vi "Process Outgoing Messages by Frame Type.vi"(0 "internal data":T1={"J1939 XNET Settings"={"XNET Database"="", "XNET Cluster"="", "CAN port"="", "Baud rate [Bd]"=0, "J1939 Network Address"=0, "Name"=0, "Termination"=0}, "j1939 queues"={"Processed Outgoing"=refnum, "Process Outgoing"=refnum, "stop notifier"=refnum, "error queue"=refnum, "active dtc"=refnum, "processed inc"=refnum}, "fgv references"={"BAM Buffer"=refnum, "CM Buffer"=refnum, "CM Gen"=refnum, "BAM Gen"=refnum, "Address Claims"=refnum, "RQST"=refnum, "scaling lut"=refnum, "data lut"=refnum, "cyclic scheduler"=refnum}, "frame in"="", "frame out"="", "timing"={"tb to j1939 queue timeout"=100, "j1939 to tb queue timeout"=100, "dtc loop period (ms)"=100, "CAN in loop period (ms)"=100, "process incoming queue timeout (ms)"=100, "Outgoing Write Decimation"=0, "process outgoing loop rate (ms)"=0, "periodic outgoing queue timeout (ms)"=10, "CAN out queue timeout (ms)"=100}}, 5 "Output Array":T14[](array[typedef]) {"Identifier" format="%08x"}, 11 "error in":errorcluster) -> (13 "Message Errors":errorcluster, 15 "System Error":errorcluster)   [LabVIEW 2013, in "J1939.lvlib"]
uses:
  J1939.lvlib
  API Types/CAN Outgoing Message Cluster.ctl
  API Types/Internal Data.ctl
  API Types/XNET Settings.ctl
  API Types/Setup Information Cluster.ctl
  API Types/Convert DTCs Cluster.ctl
  <vilib>/xnet/xnet.llb/XNET Frame CAN.ctl
  <vilib>/xnet/xnet.llb/XNET Frame Type CAN.ctl
  TP/TP List References.ctl
  BAM/BAM Buffer Connections List_Ref.ctl
  Connection Mode/Connection Mode Generation Connection Ref.ctl
  BAM/BAM Generation Connections List_Ref.ctl
  LUTs/J1939 Address Table Reference.ctl
  RQST/RQST Lookup Table Reference.ctl
  LUTs/J1939 Conversion Lookup Table Reference.ctl
  LUTs/J1939 Data Lookup Table Reference.ctl
  LUTs/Cyclic Frame Scheduler Lut Reference.ctl
  Configuration/TypeDefs/timing configuration.ctl
  TP/TP Connections List State.ctl
  BAM/BAM Generation Connections List_Actions.vi
  BAM/BAM Generation Create New TP Connection.vi
  Connection Mode/Connection Mode Generation Connections List_Actions.vi
  Connection Mode/Connection Mode Generation Search for Connection (Local Message).vi
  Connection Mode/Connection Mode Generation Create New TP Connection.vi
  Frame Conversion/Common Conversions.vi
  Frame Conversion/Convert CAN Arb ID to J1939 ID.vi
  Common Messages/J1939 Common Messages.vi
  Common Messages/J1939 Message TP.CM BAM.vi
  Common Messages/J1939 Message TP.DT.vi
  Common Messages/J1939 Message TP.CM RTS.vi
  Frame Conversion/Convert J1939 ID to CAN Arb ID.vi
  BAM/BAM Generation Search for Connection (Local Message).vi
panel:
  in  "Allow Any Source Address":bool=TRUE
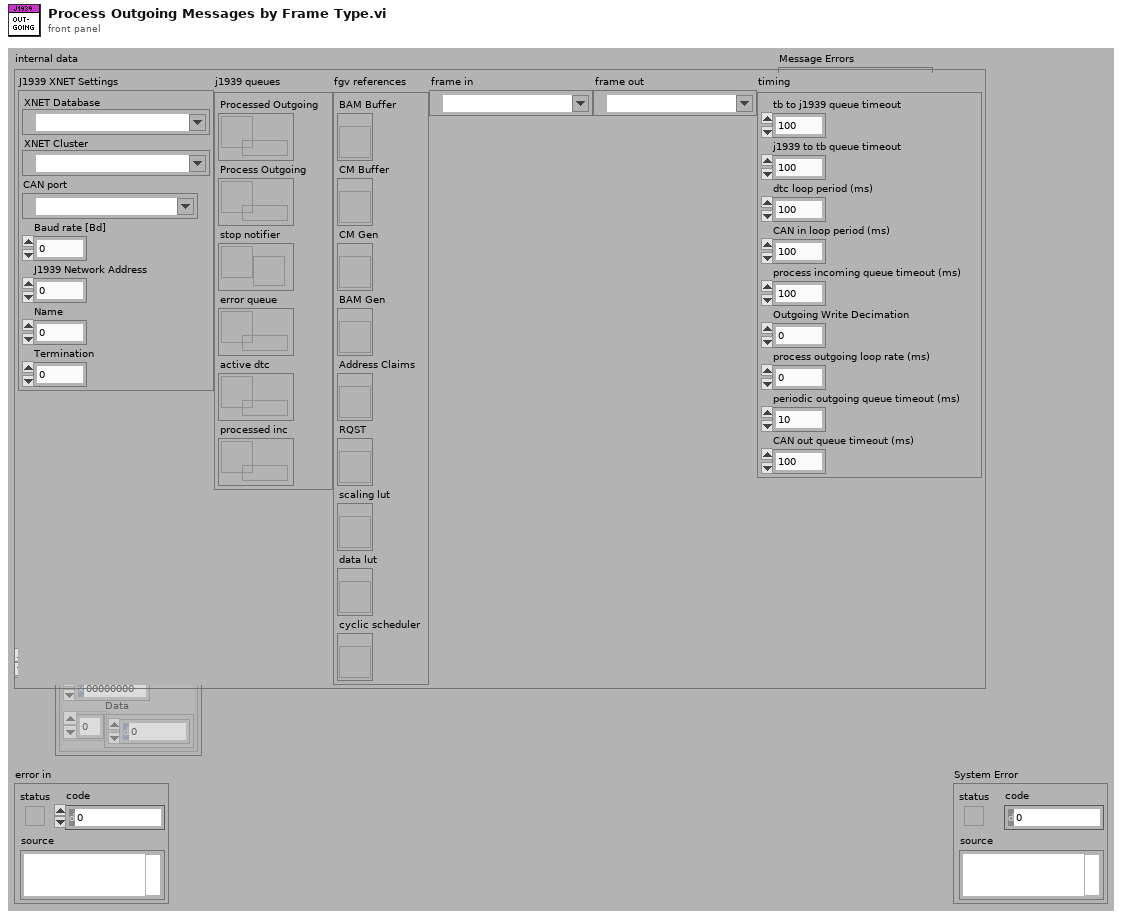
[diagram p1: front panel]
types:
  T1 = typedef "J1939.lvlib/Internal Data.ctl" = cluster{"J1939 XNET Settings":T2, "j1939 queues":T3, "fgv references":T4, "frame in":refnum<k21>, "frame out":refnum<k21>, "timing":T13}
  T2 = typedef "J1939.lvlib/XNET settings.ctl" = cluster{"XNET Database":refnum<k21>, "XNET Cluster":refnum<k21>, "CAN port":refnum<k21>, "Baud rate [Bd]":u32, "J1939 Network Address":u8, "Name":u64, "Termination":u32}
  T3 = typedef "J1939.lvlib/Setup Information Cluster.ctl" = cluster{"Processed Outgoing":refnum<queue>, "Process Outgoing":refnum<queue>, "stop notifier":refnum<notifier>, "error queue":refnum<queue>, "active dtc":refnum<queue>, "processed inc":refnum<queue>}
  T4 = typedef "J1939.lvlib/TP List References.ctl" = cluster{"BAM Buffer":T5, "CM Buffer":T5, "CM Gen":T6, "BAM Gen":T7, "Address Claims":T8, "RQST":T9, "scaling lut":T10, "data lut":T11, "cyclic scheduler":T12}
  T5 = typedef "J1939.lvlib/BAM Buffer Connections List_Ref.ctl" = refnum<vi>
  T6 = typedef "J1939.lvlib/Connection Mode Generation Connection Ref.ctl" = refnum<vi>
  T7 = typedef "J1939.lvlib/BAM Generation Connections List_Ref.ctl" = refnum<vi>
  T8 = typedef "J1939.lvlib/J1939 Address Table Reference.ctl" = refnum<vi>
  T9 = typedef "J1939.lvlib/RQST Lookup Table Reference.ctl" = refnum<vi>
  T10 = typedef "J1939.lvlib/J1939 Conversion Lookup Table Reference.ctl" = refnum<vi>
  T11 = typedef "J1939.lvlib/J1939 Data Lookup Table Reference.ctl" = refnum<vi>
  T12 = typedef "J1939.lvlib/cyclic frame scheduler lut reference.ctl" = refnum<vi>
  T13 = typedef "J1939.lvlib/timing configuration.ctl" = cluster{"tb to j1939 queue timeout":i32, "j1939 to tb queue timeout":i32, "dtc loop period (ms)":i32, "CAN in loop period (ms)":i32, "process incoming queue timeout (ms)":i32, "Outgoing Write Decimation":u32, "process outgoing loop rate (ms)":i32, "periodic outgoing queue timeout (ms)":i32, "CAN out queue timeout (ms)":i32}
  T14 = typedef "J1939.lvlib/CAN Outgoing Message Cluster.ctl" = cluster{"Identifier":u32, "Data":u8[]}
  T15 = typedef "J1939.lvlib/TP Connections List State.ctl" = enum16{"Add", "Update", "Get", "Remove", "Initialize"}
  T16 = typedef "J1939.lvlib/Outgoing Messages Frame Type.ctl" = enum16{"Standard Frame", "BAM", "Connection Mode"}
  T17 = typedef "J1939.lvlib/BAM Generation Connection Cluster.ctl" = cluster{"Total Packets":u8, "Current Packet to Generate":u8, "Packets":T14[], "Previous Time Stamp":u32, "Total Bytes":u16, "Source Address":u8}
  T18 = typedef "J1939.lvlib/Connection Mode Generation Connection Cluster.ctl" = cluster{"Total Packets":u8, "Current Packet to Generate":u8, "Packets":T14[], "Previous Time Stamp":u32, "Total Bytes":u16, "Packet Identifier [PDU S + SA]":u16, "Number of Packets to Generate":u8, "PGN":u32}
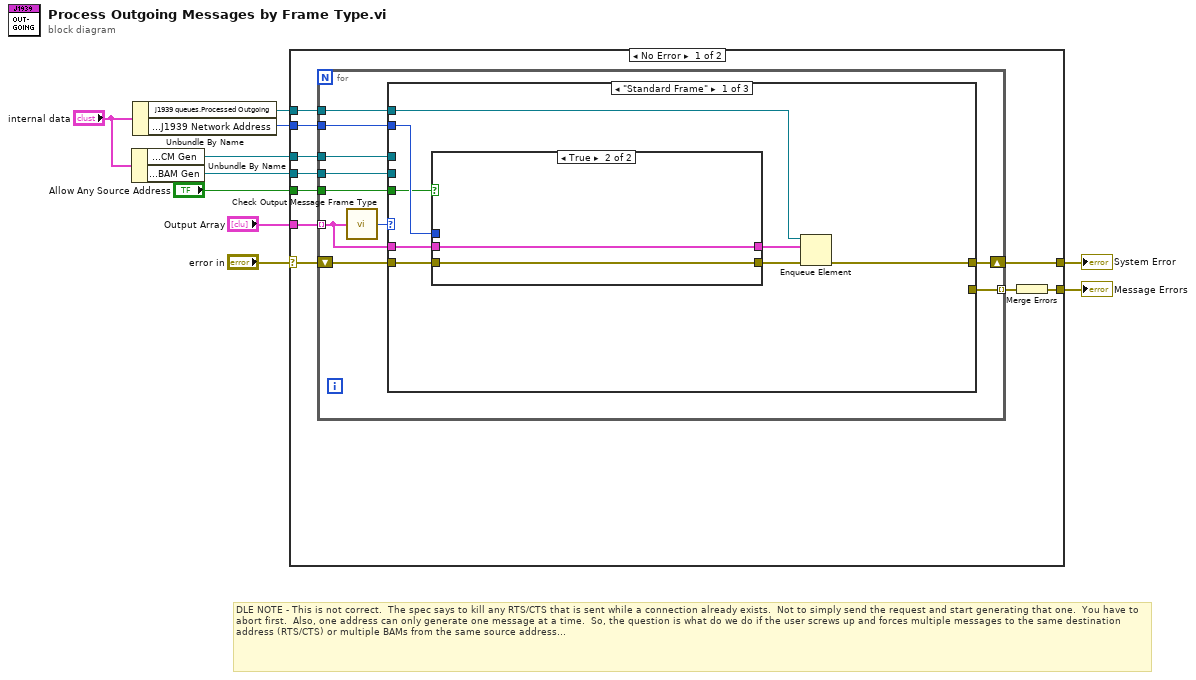
[diagram p0: block diagram]
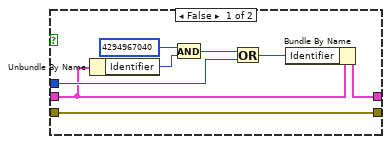
[diagram p2: hidden frame]
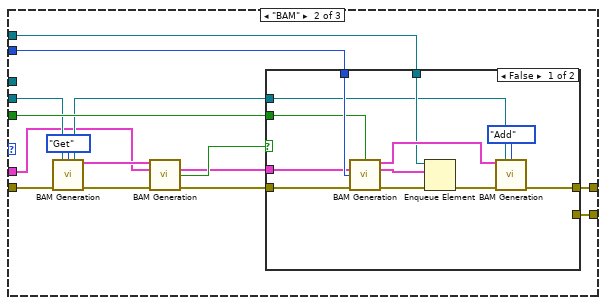
[diagram p3: hidden frame]
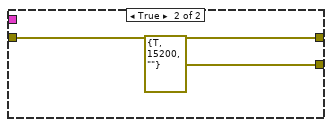
[diagram p4: hidden frame]
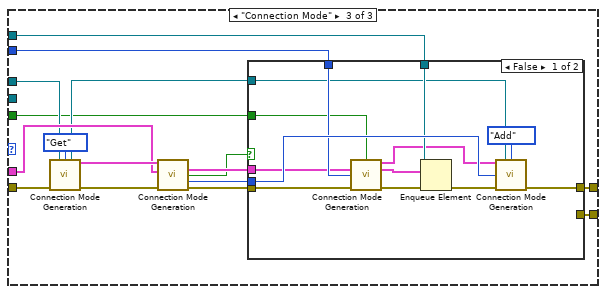
[diagram p5: hidden frame]
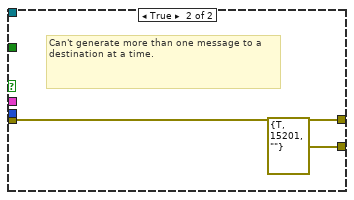
[diagram p6: hidden frame]
diagram:
  # "DLE NOTE - This is not correct.  The spec says to kill any RTS/CTS that is sent while a connection already exists.  Not to simply send the request and start generating that one.  You have to abort first.  Also, one address can only generate one message at a time.  So, the question is what do we do if the user screws up and forces multiple messages to the same destination address (RTS/CTS) or multiple BAMs from the same source address..."
  n1 = Unbundle By Name("internal data") -> ("fgv references.CM Gen"=w7:T6, "fgv references.BAM Gen"=w6:T7)
  n2 = Unbundle By Name("internal data") -> ("j1939 queues.Processed Outgoing"=w10:refnum<queue>, "J1939 XNET Settings.J1939 Network Address"=w8:u8)
  n3 = case shown="No Error" "error in" {
    selector: "error in" -> [w15 w109]
    tunnel: w10 -> [w20 _]
    tunnel: "Output Array" -> [w12 _]
    tunnel: w8 -> [w19 _]
    tunnel: w7 -> [w18 _]
    tunnel: w6 -> [w17 _]
    tunnel: "Allow Any Source Address" -> [w16 _]
    tunnel: [w11 w109] -> w3
    tunnel: [w13 w109] -> w2
    frame No Error {
      n4 = for {
        tunnel: w12 -> [w26] mode=indexing
        tunnel: w20 -> [w29]
        tunnel: w19 -> [w28]
        tunnel: w18 -> [w24]
        tunnel: w17 -> [w23]
        tunnel: w16 -> [w22]
        tunnel: [w21] -> w14 mode=indexing
        shift-right: [w30] -> w13
        shift-left: w15 -> [w25]
        n5 = call "Check Output Message Frame Type.vi"("Data to Send"=w26) -> ("Frame Type"=w27:T16)  [unwired: 14 out]
        n6 = case shown="\"Standard Frame\"" w27 {
          tunnel: w25 -> [w32 w56 w90]
          tunnel: [w37 w61 w88] -> w30
          tunnel: w28 -> [w36 w63 w86]
          tunnel: w29 -> [w38 w62 w85]
          tunnel: w26 -> [w35 w50 w83]
          tunnel: w24 -> [_ _ w82]
          tunnel: w23 -> [_ w54 _]
          tunnel: w22 -> [w31 w60 w80]
          tunnel: [_ w51 w78] -> w21
          frame "Standard Frame" {
            n7 = case shown="True" w31 {
              tunnel: w36 -> [w43 _]
              tunnel: w35 -> [w41 w48]
              tunnel: [w40 w48] -> w34
              tunnel: [w39 w47] -> w33
              tunnel: w32 -> [w39 w47]
              frame False {
                n8 = Unbundle By Name(w41) -> ("Identifier"=w44:u32)
                n9 = And(x=u32 4294967040, y=w44) -> (x .and. y?=w46:u32)
                n10 = Or(x=w46, y=w43) -> (x .or. y?=w42:u32)
                n11 = Bundle By Name(cluster=w41, "Identifier"=w42) -> (w40:T14)
              }
              frame True {
              }
            }
            n12 = Enqueue Element(queue=w38, element=w34, error in (no error)=w33) -> (error out=w37:errorcluster)  [unwired: 3 out]
          }
          frame "BAM" {
            n13 = call-poly "BAM Generation.vi"("ref in"=w54, "State"=TP_Connections_List_State."Get", "error in (no error)"=w56) -> ("ref out"=w53:T7, "Connections"=w58:T17[], "error out"=w57:errorcluster)  [unwired: 3 in, 7 out]
            n14 = call-poly "BAM Generation.vi"("Connections"=w58, "Data to Send"=w50, "error in (no error)"=w57) -> ("CAN Frame Out"=w49:T14, "Found?"=w52:bool, "error out"=w55:errorcluster)  [unwired: 1 in, 9 out]
            n15 = case shown="False" w52 {
              tunnel: w63 -> [w71 _]
              tunnel: w62 -> [w70 _]
              tunnel: [w69 w76] -> w61
              tunnel: w60 -> [w67 _]
              tunnel: w49 -> [w66 _]
              tunnel: w55 -> [w65 w76]
              tunnel: w53 -> [w64 _]
              tunnel: [_ errorcluster {"status"=TRUE, "code"=15200, "source"=""} ("error out")] -> w51
              frame False {
                n16 = call-poly "BAM Generation.vi"("Allow Any SA"=w67, "Data to Send"=w66, "Source Address"=w71, "error in (no error)"=w65) -> ("Connection Cluster"=w75:T17, "Connection Management Packet"=w68:T14, "error out"=w73:errorcluster)  [unwired: 1 in, 8 out]
                n17 = Enqueue Element(queue=w70, element=w68, error in (no error)=w73) -> (error out=w74:errorcluster)  [unwired: 3 out]
                n18 = call-poly "BAM Generation.vi"("Connection Cluster"=w75, "ref in"=w64, "State"=TP_Connections_List_State."Add", "error in (no error)"=w74) -> ("error out"=w69:errorcluster)  [unwired: 1 in, 10 out]
              }
              frame True {
              }
            }
          }
          frame "Connection Mode" {
            n19 = call-poly "Connection Mode Generation.vi"("ref in"=w82, "State"=TP_Connections_List_State."Get", "error in (no error)"=w90) -> ("ref out"=w81:T6, "Connections"=w91:T18[], "error out"=w92:errorcluster)  [unwired: 2 in, 8 out]
            n20 = call-poly "Connection Mode Generation.vi"("Connections"=w91, "Data to Send"=w83, "error in (no error)"=w92) -> ("CAN Frame Out"=w84:T14, "Found?"=w79:bool, "Index"=w87:i32, "error out"=w89:errorcluster)  [unwired: 1 in, 8 out]
            n21 = case shown="False" w79 {
              tunnel: w89 -> [w106 w107]
              tunnel: [w105 w107] -> w88
              tunnel: w87 -> [w104 _]
              tunnel: w86 -> [w103 _]
              tunnel: w85 -> [w100 _]
              tunnel: w84 -> [w98 _]
              tunnel: w81 -> [w97 _]
              tunnel: w80 -> [w95 _]
              tunnel: [_ errorcluster {"status"=TRUE, "code"=15201, "source"=""} ("error out")] -> w78
              frame False {
                n22 = call-poly "Connection Mode Generation.vi"("Allow Any SA"=w95, "Data to Send"=w98, "Source Address"=w103, "error in (no error)"=w106) -> ("Connections Cluster"=w99:T18, "Connection Management Packet"=w96:T14, "error out"=w102:errorcluster)  [unwired: 9 out]
                n23 = Enqueue Element(queue=w100, element=w96, error in (no error)=w102) -> (error out=w101:errorcluster)  [unwired: 3 out]
                n24 = call-poly "Connection Mode Generation.vi"("Connection Cluster"=w99, "ref in"=w97, "State"=TP_Connections_List_State."Add" ("f"), "index"=w104, "error in (no error)"=w101) -> ("error out"=w105:errorcluster)  [unwired: 10 out]
              }
              frame True {
                # "Can't generate more than one message to a destination at a time."
              }
            }
          }
        }
      }
      n25 = Merge Errors(w14) -> (w11:errorcluster)
    }
    frame Error {
    }
  }
  "Message Errors" <- w3
  "System Error" <- w2
